vi "AllTests.vi"(0 "VI in":refnum<vi>, 1 "Label":string, 11 "error in (no error)":errorcluster) -> (4 "VI out":refnum<vi>, 15 "error out":errorcluster)   [LabVIEW 2016, in "Drona Test.lvlib"]
uses:
  Drona Test.lvlib
  <vilib>/addons/_JKI Toolkits/Caraya/classes/Assert/Assert Not Error.vi
  <vilib>/addons/_JKI Toolkits/Caraya/classes/Assert/Assert.lvclass
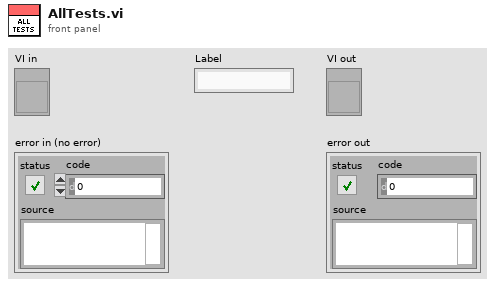
[diagram p1: front panel]
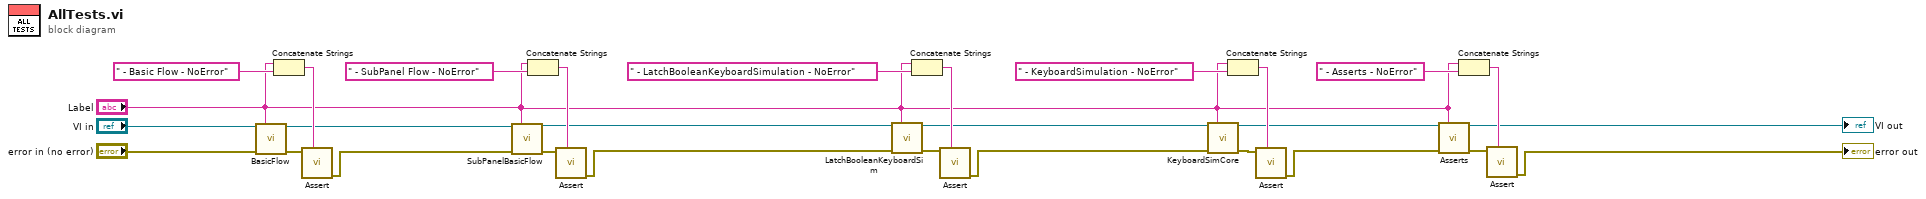
[diagram p0: block diagram]
diagram:
  n1 = call "BasicFlow.vi"("VI Reference In"="VI in", "Label (VI Title)"="Label", "error in (no error)"="error in (no error)") -> ("VI Reference Out"=w24:refnum<vi>, "error out"=w23:errorcluster)  [unwired: 11 in]
  n2 = Concatenate Strings("Label", " - Basic Flow - NoError" ("string")) -> (w25:string)
  n3 = call-poly <vilib>:"Assert.vi"("Label"=w25, "Not Error?"=w23) -> ("error out"=w22:errorcluster)  [unwired: 9 in]
  n4 = call "SubPanelBasicFlow.vi"("VI Reference In"=w24, "Label (VI Title)"="Label", "error in (no error)"=w22) -> ("VI Reference Out"=w14:refnum<vi>, "error out"=w19:errorcluster)  [unwired: 11 in]
  n5 = Concatenate Strings("Label", " - SubPanel Flow - NoError" ("string")) -> (w21:string)
  n6 = call-poly <vilib>:"Assert.vi"("Label"=w21, "Not Error?"=w19) -> ("error out"=w18:errorcluster)  [unwired: 9 in]
  n7 = call "LatchBooleanKeyboardSim.vi"("VI Reference In"=w14, "Label (VI Title)"="Label", "error in (no error)"=w18) -> ("VI Reference Out"=w11:refnum<vi>, "error out"=w15:errorcluster)  [unwired: 11 in]
  n8 = Concatenate Strings("Label", " - LatchBooleanKeyboardSimulation - NoError" ("string")) -> (w16:string)
  n9 = call-poly <vilib>:"Assert.vi"("Label"=w16, "Not Error?"=w15) -> ("error out"=w9:errorcluster)  [unwired: 9 in]
  n10 = call "KeyboardSimCore.vi"("VI Reference In"=w11, "Label (VI Title)"="Label", "error in (no error)"=w9) -> ("VI Reference Out"=w5:refnum<vi>, "error out"=w10:errorcluster)  [unwired: 11 in]
  n11 = Concatenate Strings("Label", " - KeyboardSimulation - NoError" ("string")) -> (w13:string)
  n12 = call-poly <vilib>:"Assert.vi"("Label"=w13, "Not Error?"=w10) -> ("error out"=w4:errorcluster)  [unwired: 9 in]
  n13 = call "Asserts.vi"("VI Reference In"=w5, "Label (VI Title)"="Label", "error in (no error)"=w4) -> ("VI Reference Out"=→"VI out":refnum<vi>, "error out"=w8:errorcluster)  [unwired: 11 in]
  n14 = Concatenate Strings("Label", " - Asserts - NoError" ("string")) -> (w6:string)
  n15 = call-poly <vilib>:"Assert.vi"("Label"=w6, "Not Error?"=w8) -> ("error out"=→"error out":errorcluster)  [unwired: 9 in]
